vi "Pull Info From XNET Database.vi"(8 "error in":errorcluster, 10 "Frame Configuration":T1 {"CRC"."Data Type" items=["Signed", "Unsigned", "IEEE Float"]; "Rolling Counter"."Data Type" items=["Signed", "Unsigned", "IEEE Float"]; "Input Channels"."Data Type" items=["Signed", "Unsigned", "IEEE Float"]}, 11 "Parent Ref":T4=18446744073709551615 format="%.0x") -> (0 "error out":errorcluster, 2 "Frame Configuration":T1 {"CRC"."Data Type" items=["Signed", "Unsigned", "IEEE Float"]; "Rolling Counter"."Data Type" items=["Signed", "Unsigned", "IEEE Float"]; "Input Channels"."Data Type" items=["Signed", "Unsigned", "IEEE Float"]}, 3 "Item Ref out":T4 format="%.0x")   [LabVIEW 2015, in "Protection and Rolling Counter Addon System Explorer.lvlib"]
uses:
  Protection and Rolling Counter Addon System Explorer.lvlib
  Shared/Types/FrameConfiguration.ctl
  Shared/Types/InputChannelConfiguration.ctl
  Shared/Types/Protection Type.ctl
  <vilib>/NI Veristand/Custom Device API/Custom Device Item Ref.ctl
  NationalInstruments.VeriStand.SystemStorage
  NationalInstruments.VeriStand
  <vilib>/NI Veristand/Custom Device API/Custom Device API.lvlib
  <vilib>/NI Veristand/Custom Device Tools/Custom Device Utility Library/Custom Device Utility Library.lvlib
  <resource>/objmgr/xnet.rc
  Shared/Protection and Rolling Counter Addon Shared.lvlib
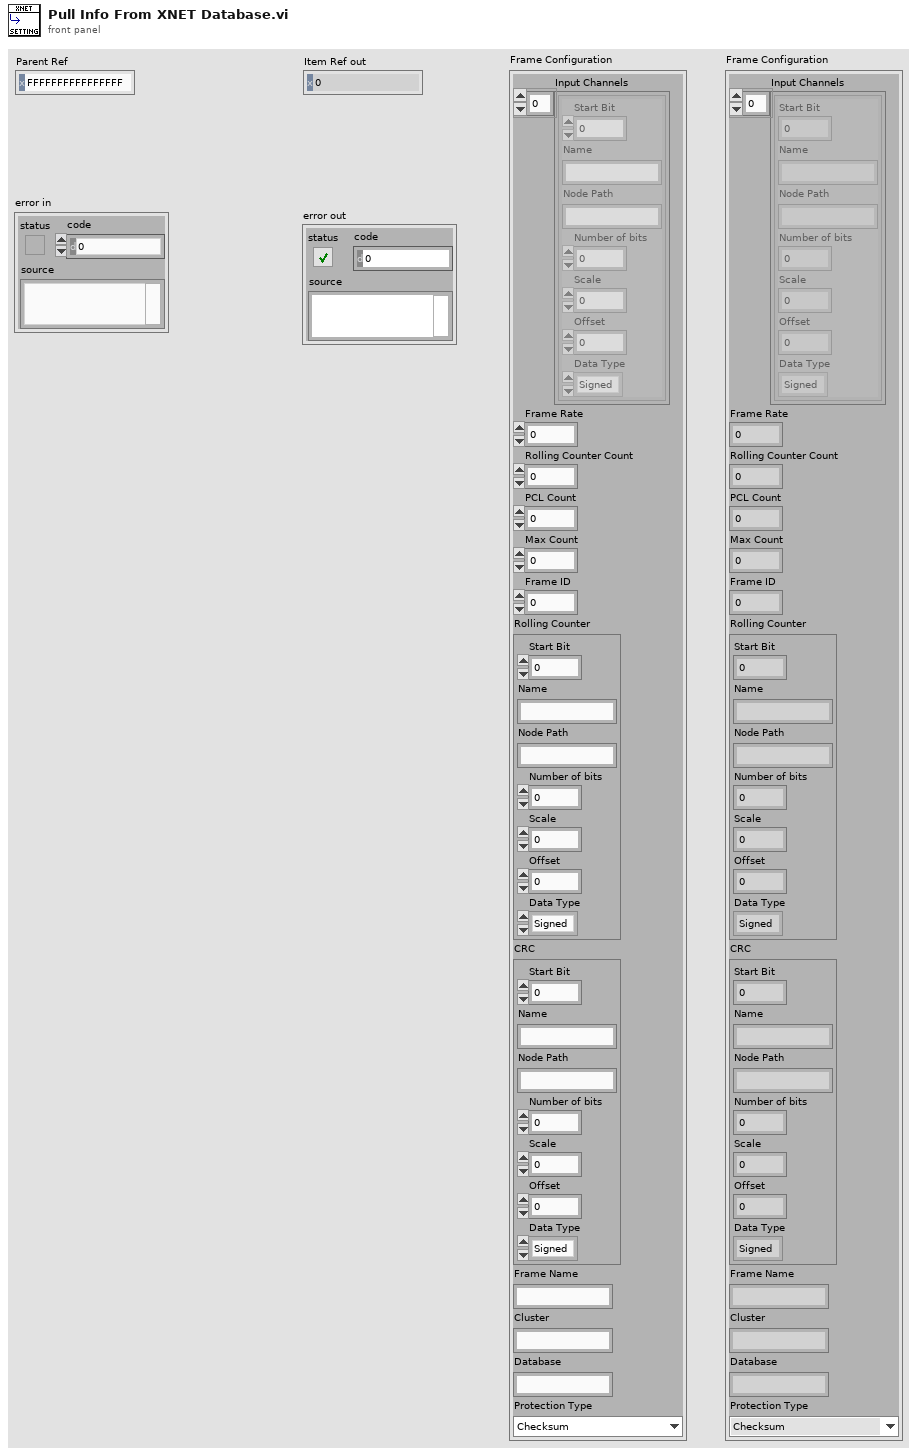
[diagram p1: front panel]
types:
  T1 = typedef "Protection and Rolling Counter Addon Shared.lvlib/FrameConfiguration.ctl" = cluster{"Input Channels":T2[], "Frame Rate":dbl, "Rolling Counter Count":dbl, "PCL Count":u64, "Max Count":dbl, "Frame ID":u32, "Rolling Counter":T2, "CRC":T2, "Frame Name":string, "Cluster":string, "Database":string, "Protection Type":T3}
  T2 = typedef "Protection and Rolling Counter Addon Shared.lvlib/InputChannelConfiguration.ctl" = cluster{"Start Bit":i32, "Name":string, "Node Path":string, "Number of bits":i32, "Scale":dbl, "Offset":dbl, "Data Type":u32}
  T3 = typedef "Protection and Rolling Counter Addon Shared.lvlib/Protection Type.ctl" = enum16{"Checksum", "CRC", "None (Counter Only)"}
  T4 = typedef "Custom Device API.lvlib/Custom Device Item Ref.ctl" = u64
  T5 = typedef "Custom Device API.lvlib/Custom Device Pointer.ctl" = refnum<k24>
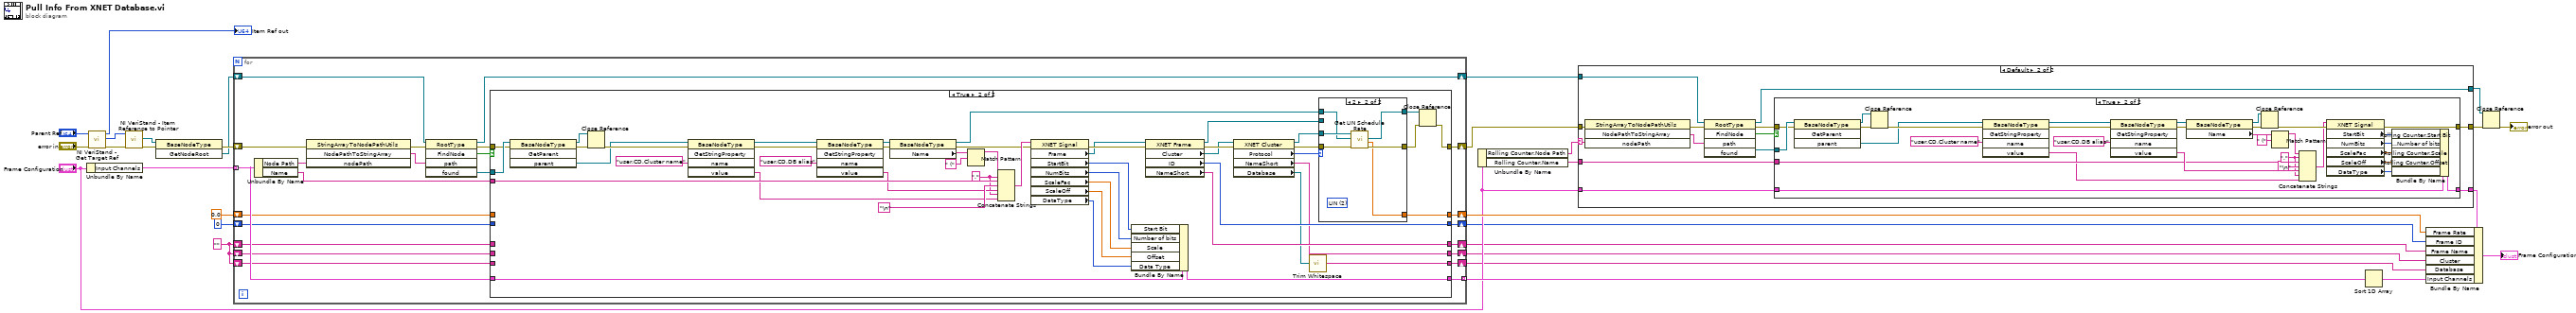
[diagram p0: block diagram]
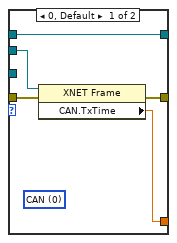
[diagram p3: hidden frame]
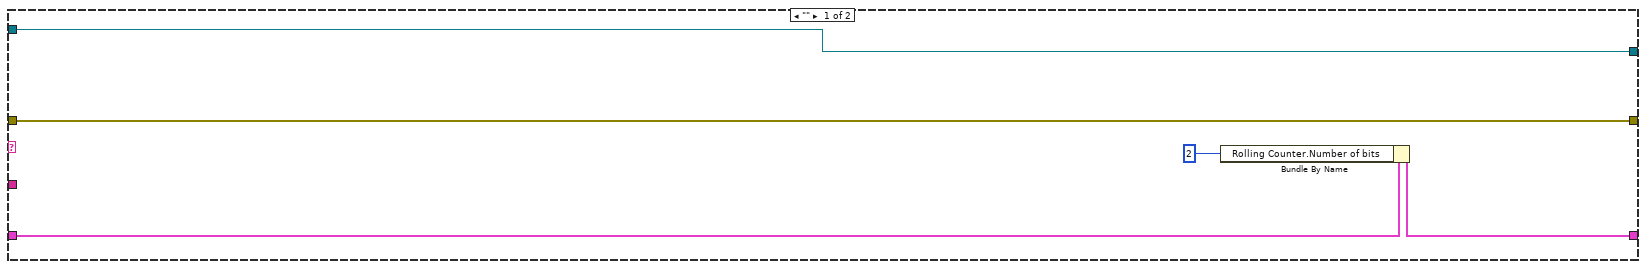
[diagram p4: hidden frame]
diagram:
  w7 = "" ("NameShort")
  n1 = Unbundle By Name("Frame Configuration") -> ("Input Channels"=w26:T2[])
  n2 = call <vilib>:"NI VeriStand - Get Target Ref.vi"("error in"="error in", "Item Ref in"="Parent Ref") -> ("error out"=w27:errorcluster, "Target Ref"=w28:T4, "Item Ref out"=→"Item Ref out":T4)  [unwired: 6 in, 1 out]
  n3 = call <vilib>:"NI VeriStand - Item Reference to Pointer.vi"("error in (no error)"=w27, "Item Ref in"=w28) -> ("error out"=w22:errorcluster, "Node Pointer"=w23:T5)  [unwired: 6 in, 2 out]
  n4 = invoke class="BaseNodeType" method="GetNodeRoot"(reference=w23, error in=w22) -> (error out=w21:errorcluster, "GetNodeRoot"=w2:refnum<k24>)  [unwired: 1 in, 1 out]
  n5 = for {
    shift-right: [w49] -> w14
    shift-left: w21 -> [w53]
    tunnel: w26 -> [w43] mode=indexing
    tunnel: [w42] -> w20 mode=indexing
    shift-right: [w41] -> w16
    shift-left: 0.0 ("CAN.TxTime") -> [w40]
    shift-right: [w39] -> w8
    shift-left: u32 0 ("ID") -> [w38]
    shift-right: [w37] -> w4
    shift-left: w7 -> [w36]
    shift-right: [w35] -> w5
    shift-left: w7 -> [w33]
    shift-right: [w34] -> w6
    shift-left: w7 -> [w32]
    shift-right: [w31] -> w1
    shift-left: w2 -> [w47]
    n6 = Unbundle By Name(w43) -> ("Node Path"=w48:string, "Name"=w44:string)
    n7 = invoke class="StringArrayToNodePathUtils" method="NodePathToStringArray"(error in=w53, "nodePath"=w48) -> (error out=w52:errorcluster, "NodePathToStringArray"=w46:string[])  [unwired: 2 in, 2 out]
    n8 = invoke class="RootType" method="FindNode"(reference=w47, error in=w52, "path"=w46) -> (reference out=w31:refnum<k24>, error out=w45:errorcluster, "FindNode"=w50:bool, "found"=w51:refnum<k24>)  [unwired: 2 in, 1 out]
    n9 = case shown="True" w50 {
      tunnel: w45 -> [w60 w106]
      tunnel: w51 -> [_ w107]
      tunnel: [w60 w61] -> w49
      tunnel: w44 -> [_ w104]
      tunnel: w43 -> [w59 w103]
      tunnel: [w59 w99] -> w42
      tunnel: [w58 w69] -> w41
      tunnel: w40 -> [w58 _]
      tunnel: [w57 w90] -> w39
      tunnel: w38 -> [w57 _]
      tunnel: [w56 w89] -> w37
      tunnel: w36 -> [w56 _]
      tunnel: [w55 w62] -> w35
      tunnel: [w54 w88] -> w34
      tunnel: w33 -> [w55 _]
      tunnel: w32 -> [w54 _]
      frame False {
      }
      frame True {
        w77 = "." ("string")
        n10 = invoke class="BaseNodeType" method="GetParent"(reference=w107, error in=w106) -> (reference out=w95:refnum<k24>, error out=w96:errorcluster, "parent"=w80:refnum<k24>)  [unwired: 2 in, 1 out]
        n11 = Close Reference(reference=w95, error in (no error)=w96) -> (error out=w82:errorcluster)
        n12 = invoke class="BaseNodeType" method="GetStringProperty"(reference=w80, error in=w82, "name"="user.CD.Cluster name") -> (reference out=w79:refnum<k24>, error out=w81:errorcluster, "value"=w76:string)  [unwired: 2 in, 2 out]
        n13 = invoke class="BaseNodeType" method="GetStringProperty"(reference=w79, error in=w81, "name"="user.CD.DB alias") -> (reference out=w84:refnum<k24>, error out=w94:errorcluster, "value"=w78:string)  [unwired: 2 in, 2 out]
        n14 = property class="BaseNodeType"(reference=w84, error in=w94) -> (reference out=w66:refnum<k24>, error out=w67:errorcluster, "Name"=w93:string)
        n15 = Match Pattern(string=w93, regular expression=" (") -> (before substring=w87:string)  [unwired: 1 in, 3 out]
        n16 = Concatenate Strings(w87, w77, w104, "\n", w78, w77, w76) -> (w75:string)
        n17 = property class="XNET Signal"(reference=w75, error in=w67) -> (error out=w97:errorcluster, "Frame"=w85:refnum<k21>, "StartBit"=w98:u32, "NumBits"=w102:u32, "ScaleFac"=w100:dbl, "ScaleOff"=w101:dbl, "DataType"=w91:u32)  [unwired: 1 out]
        n18 = Bundle By Name(cluster=w103, "Start Bit"=w98, "Number of bits"=w102, "Scale"=w100, "Offset"=w101, "Data Type"=w91) -> (w99:T2)
        n19 = property class="XNET Frame"(reference=w85, error in=w97) -> (reference out=w68:refnum<k21>, error out=w74:errorcluster, "Cluster"=w73:refnum<k21>, "ID"=w90:u32, "NameShort"=w89:string)
        n20 = property class="XNET Cluster"(reference=w73, error in=w74) -> (reference out=w71:refnum<k21>, error out=w70:errorcluster, "Protocol"=w72:u32, "NameShort"=w62:string, "Database"=w63:refnum<k21>)
        n21 = call <vilib>:"Trim Whitespace.vi"("string"=w63) -> ("trimmed string"=w88:string)  [unwired: 1 in]
        n22 = case shown="2" w72 {
          tunnel: w71 -> [_ w116]
          tunnel: [w108 w117] -> w64
          tunnel: w70 -> [w112 w118]
          tunnel: [w111 w114] -> w69
          tunnel: w68 -> [w110 _]
          tunnel: w66 -> [w109 w115]
          tunnel: [w109 w113] -> w65
          frame 0, Default {
            (unwired) u32 0 items=["CAN", "FlexRay", "LIN"] ("Protocol")
            n23 = property class="XNET Frame"(reference=w110, error in=w112) -> (error out=w108:errorcluster, "CAN.TxTime"=w111:dbl)  [unwired: 1 out]
          }
          frame 2 {
            (unwired) u32 2 items=["CAN", "FlexRay", "LIN"] ("Protocol")
            n24 = call "Get LIN Schedule Rate.vi"("error in (no error)"=w118, "Frame Ref"=w115, "XNET Cluster"=w116) -> ("error out"=w117:errorcluster, "Rate"=w114:dbl, "Frame Ref out"=w113:refnum<k24>)  [unwired: 5 in, 1 out]
          }
        }
        n25 = Close Reference(reference=w65, error in (no error)=w64) -> (error out=w61:errorcluster)
      }
    }
  }
  n26 = Unbundle By Name("Frame Configuration") -> ("Rolling Counter.Node Path"=w10:string, "Rolling Counter.Name"=w15:string)
  n27 = case shown="Default" w10 {
    selector: w10 -> [_ w125]
    tunnel: w15 -> [_ w131]
    tunnel: w1 -> [w119 w130]
    tunnel: w14 -> [w123 w129]
    tunnel: [w123 w128] -> w13
    tunnel: "Frame Configuration" -> [w122 w127]
    tunnel: [w121 w126] -> w11
    tunnel: [w119 w124] -> w3
    frame "" {
      n28 = Bundle By Name(cluster=w122, "Rolling Counter.Number of bits"=u32 2 ("Rolling Counter Length")) -> (w121:T1)
    }
    frame Default {
      n29 = invoke class="StringArrayToNodePathUtils" method="NodePathToStringArray"(error in=w129, "nodePath"=w125) -> (error out=w136:errorcluster, "NodePathToStringArray"=w133:string[])  [unwired: 2 in, 2 out]
      n30 = invoke class="RootType" method="FindNode"(reference=w130, error in=w136, "path"=w133) -> (reference out=w124:refnum<k24>, error out=w132:errorcluster, "FindNode"=w134:bool, "found"=w135:refnum<k24>)  [unwired: 2 in, 1 out]
      n31 = case shown="True" w134 {
        tunnel: w132 -> [w138 w169]
        tunnel: w135 -> [_ w170]
        tunnel: [w138 w158] -> w128
        tunnel: w131 -> [_ w165]
        tunnel: w127 -> [w137 w164]
        tunnel: [w137 w162] -> w126
        frame False {
        }
        frame True {
          w141 = "." ("string")
          n32 = invoke class="BaseNodeType" method="GetParent"(reference=w170, error in=w169) -> (reference out=w159:refnum<k24>, error out=w160:errorcluster, "parent"=w143:refnum<k24>)  [unwired: 2 in, 1 out]
          n33 = Close Reference(reference=w159, error in (no error)=w160) -> (error out=w145:errorcluster)
          n34 = invoke class="BaseNodeType" method="GetStringProperty"(reference=w143, error in=w145, "name"="user.CD.Cluster name") -> (reference out=w142:refnum<k24>, error out=w144:errorcluster, "value"=w140:string)  [unwired: 2 in, 2 out]
          n35 = invoke class="BaseNodeType" method="GetStringProperty"(reference=w142, error in=w144, "name"="user.CD.DB alias") -> (reference out=w155:refnum<k24>, error out=w157:errorcluster, "value"=w166:string)  [unwired: 2 in, 2 out]
          n36 = property class="BaseNodeType"(reference=w155, error in=w157) -> (reference out=w154:refnum<k24>, error out=w156:errorcluster, "Name"=w152:string)
          n37 = Close Reference(reference=w154, error in (no error)=w156) -> (error out=w161:errorcluster)
          n38 = Match Pattern(string=w152, regular expression=" (") -> (before substring=w151:string)  [unwired: 1 in, 3 out]
          n39 = Concatenate Strings(w151, w141, w165, "\n", w166, w141, w140) -> (w139:string)
          n40 = property class="XNET Signal"(reference=w139, error in=w161) -> (error out=w158:errorcluster, "StartBit"=w163:u32, "NumBits"=w150:u32, "ScaleFac"=w149:dbl, "ScaleOff"=w148:dbl, "DataType"=w147:u32)  [unwired: 1 out]
          n41 = Bundle By Name(cluster=w164, "Rolling Counter.Start Bit"=w163, "Rolling Counter.Number of bits"=w150, "Rolling Counter.Scale"=w149, "Rolling Counter.Offset"=w148, "Rolling Counter.Data Type"=w147) -> (w162:T1)
        }
      }
    }
  }
  n42 = Sort 1D Array(array=w20) -> (sorted array=w18:T2[])
  n43 = Bundle By Name(cluster=w11, "Frame Rate"=w16, "Frame ID"=w8, "Frame Name"=w4, "Cluster"=w5, "Database"=w6, "Input Channels"=w18) -> (→"Frame Configuration":T1)
  n44 = Close Reference(reference=w3, error in (no error)=w13) -> (error out=→"error out":errorcluster)
